vi "Orion PDU Read Status.vi"(8 "error in (no error)":errorcluster, 10 "Address":string, 11 "client handle":T1) -> (0 "error out":errorcluster, 1 "current":dbl, 2 "states":bool[](array[boolean]), 3 "client handle out":T1)   [LabVIEW 2022 SP3, in "Orion PDU.lvclass"]
uses:
  Orion PDU.lvclass
  Orion PDU.lvclass/Orion PDU.ctl
  <vilib>/httpClient/LabVIEWHTTPClient.lvlib
  <vilib>/httpClient/POSTBuffer.vi
  <vilib>/regexp/Match Regular Expression.xnode
  <vilib>/httpClient/ClientHandle.ctl
panel:
  out "body":string
  out "headers":string
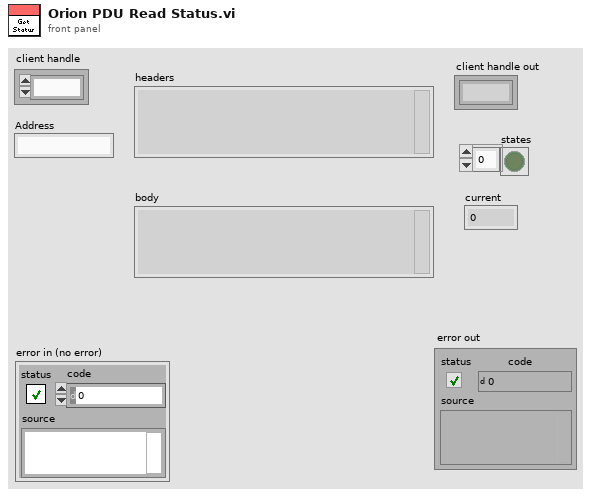
[diagram p1: front panel]
types:
  T1 = typedef "LabVIEWHTTPClient.lvlib/ClientHandle.ctl" = refnum<k1>
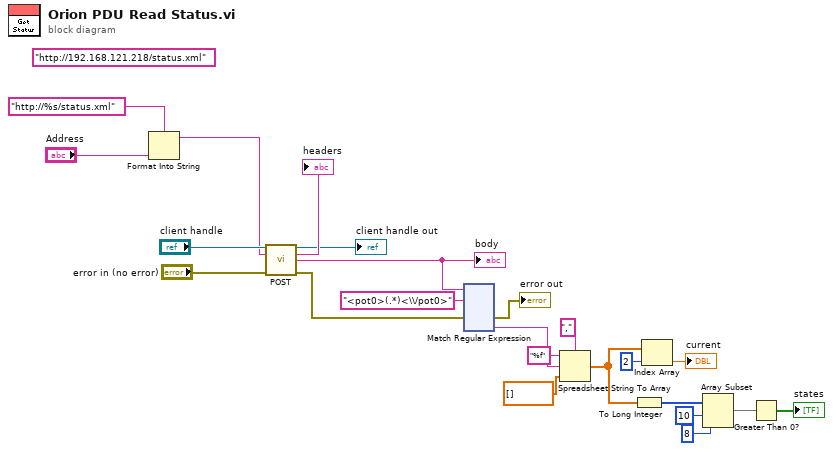
[diagram p0: block diagram]
diagram:
  (unwired) "http://192.168.121.218/status.xml"
  n1 = Format Into String(format string="http://%s/status.xml", "Address") -> (resulting string=w2:string)  [unwired: 2 in, 1 out]
  n2 = call-poly <vilib>:"POST.vi"("client handle"="client handle", "url"=w2, "error in (no error)"="error in (no error)") -> ("client handle out"=→"client handle out":T1, "headers"=→"headers":string, "body"=w8:string, "error out"=w7:errorcluster)  [unwired: 9 in]
  "body" <- w8
  n3 = xnode "Match Regular Expression"("input string"=w8, "regular expression"="<pot0>(.*)<\\/pot0>", "error in"=w7) -> ("error out"=→"error out":errorcluster, "submatch 1"=w22:string)  [unwired: 3 in, 4 out]
  n4 = Spreadsheet String To Array(delimiter (Tab)=",", format string="%f", spreadsheet string=w22, array type (2D Dbl)=dbl[] []) -> (array=w14:dbl[])
  n5 = To Long Integer(number=w14) -> (32bit integer=w18:i32[])
  n6 = Index Array(array=w14, index=2) -> (element=→"current":dbl)
  n7 = Array Subset(array=w18, index=10, length=8) -> (w15:i32[])
  n8 = Greater Than 0?(x=w15) -> (x > 0?=→"states":bool[])
